vi "Set_Control_Values_by_Index_(Sgnl)_ExpTab.vi"(7 "Control References":refnum<vi>[](array[refnum]), 8 "error in (no error)":errorcluster, 9 "appended array":variant[](array[variant]), 11 "VI Refnum":refnum<vi>) -> (0 "error out":errorcluster, 3 "VI Refnum":refnum<vi>)   [LabVIEW 2015]
panel:
  out "appended array 2":variant[](array[variant])
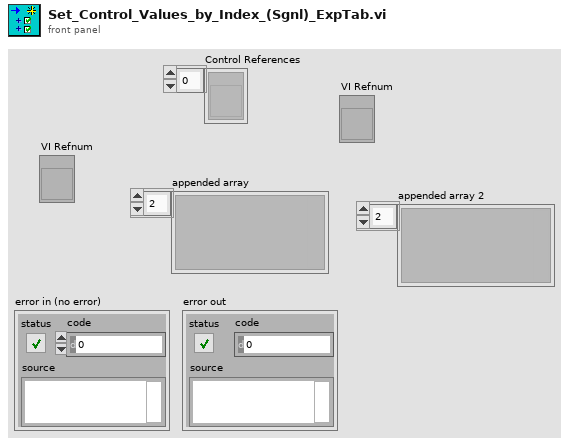
[diagram p1: front panel]
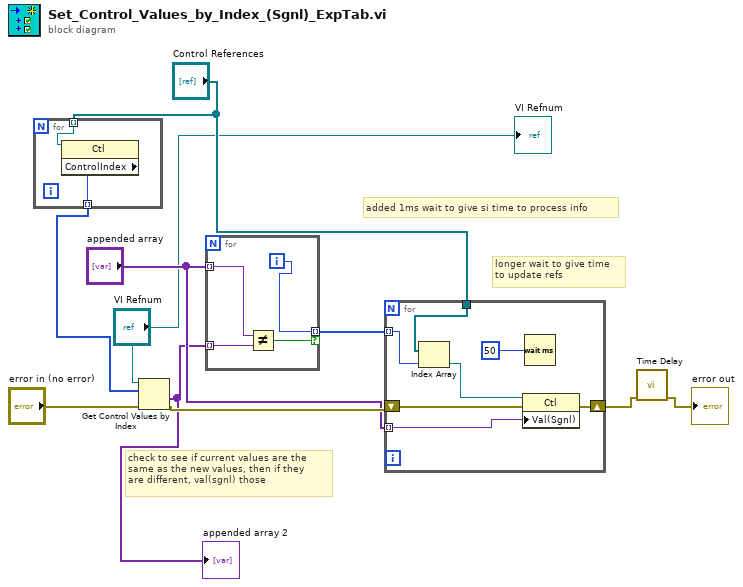
[diagram p0: block diagram]
diagram:
  # "longer wait to give time\nto update refs"
  # "check to see if current values are the \nsame as the new values, then if they\nare different, val(sgnl) those"
  # "added 1ms wait to give si time to process info"
  n1 = for {
    tunnel: "Control References" -> [w12] mode=indexing
    tunnel: [w11] -> w7 mode=indexing
    n2 = property class="Ctl"(reference=w12) -> ("ControlIndex"=w11:i32)  [unwired: 1 in, 2 out]
  }
  n3 = Get Control Values by Index(0:"VI Refnum", 1:w7, 3:"error in (no error)") -> (10:w3:variant[], 11:w6:errorcluster)
  "appended array 2" <- w3
  n4 = for {
    tunnel: "appended array" -> [w16] mode=indexing
    tunnel: w3 -> [w15] mode=indexing
    tunnel: [w13] -> w10 mode=indexing if=w14
    i -> [w13]
    n5 = Not Equal?(x=w16, y=w15) -> (x != y?=w14:bool)
  }
  n6 = for {
    tunnel: w10 -> [w21] mode=indexing
    shift-right: [w23] -> w2
    shift-left: w6 -> [w18]
    tunnel: "Control References" -> [w22]
    tunnel: "appended array" -> [w17] mode=indexing
    n7 = Index Array(array=w22, index=w21) -> (element=w19:refnum<vi>)
    n8 = property class="Ctl"(reference=w19, error in=w18, "Val(Sgnl)"=w17) -> (error out=w23:errorcluster)  [unwired: 1 out]
    n9 = Wait (ms)(milliseconds to wait=50) -> ()  [unwired: 1 out]
  }
  n10 = call "Time Delay"("error in (no error)"=w2) -> ("error out"=→"error out":errorcluster)  [unwired: 10 in]
  "VI Refnum" <- "VI Refnum"
